vi "Proyecto Autotrónica.vi"() -> ()   [LabVIEW 2025]
uses:
  <vilib>/MakerHub/LINX/Public/Peripherals/Analog/Analog Read 1 Chan.vi
  <vilib>/MakerHub/LINX/Public/Peripherals/Digital/Digital Read 1 Chan.vi
  <vilib>/MakerHub/LINX/Public/Peripherals/Analog/Analog Read N Chans.vi
  <vilib>/MakerHub/LINX/Public/Peripherals/Digital/Digital Read N Chans.vi
  <vilib>/MakerHub/LINX/Private/Local IO/LinxAnalogRead.vi
  <vilib>/MakerHub/LINX/Public/Utilities/Check Channel.vi
  <vilib>/MakerHub/LINX/Private/Local IO/LinxDigitalRead.vi
  <vilib>/MakerHub/LINX/Public/Utilities/Open Serial.vi
  <vilib>/MakerHub/LINX/Private/Utilties/Generate Error.vi
  <vilib>/express/express shared/transition.llb/Dynamic To Waveform Array.vi
  <vilib>/express/express signal manip/GetorSetDDTAttributes/Set DDT Attributes/SetT0.vi
  <vilib>/express/express shared/transition.llb/Waveform Array To Dynamic.vi
  <vilib>/express/express signal manip/GetorSetDDTAttributes/Set DDT Attributes/Set DDT Properties.xnode
  <vilib>/MakerHub/LINX/LMH-LINX.lvlib
panel:
  out "?":bool
  out "?":bool
  out "?":bool
  out "?":bool
  out "Llave":bool
  out "Velocidad (MPH)":dbl
  in  "Serial Port":refnum<visa-resource-name>="N/A"
  out "TPMS":T1(graph)
  in  "stop":bool
  out "P3":bool
  out "P2":bool
  out "P1":bool
  out "Rueda RR ( BAR)":dbl
  out "Rueda RR  (PSI)":dbl
  out "Rueda LR (BAR)":dbl
  out "Rueda LR  (PSI)":dbl
  out "Rueda RF  (BAR)":dbl
  out "Rueda LF  (BAR)":dbl
  out "Rueda RF  (PSI)":dbl
  out "Rueda LF (PSI)":dbl
  out "Velocidad (km/h)":dbl(knob) scale=0.0..220.0
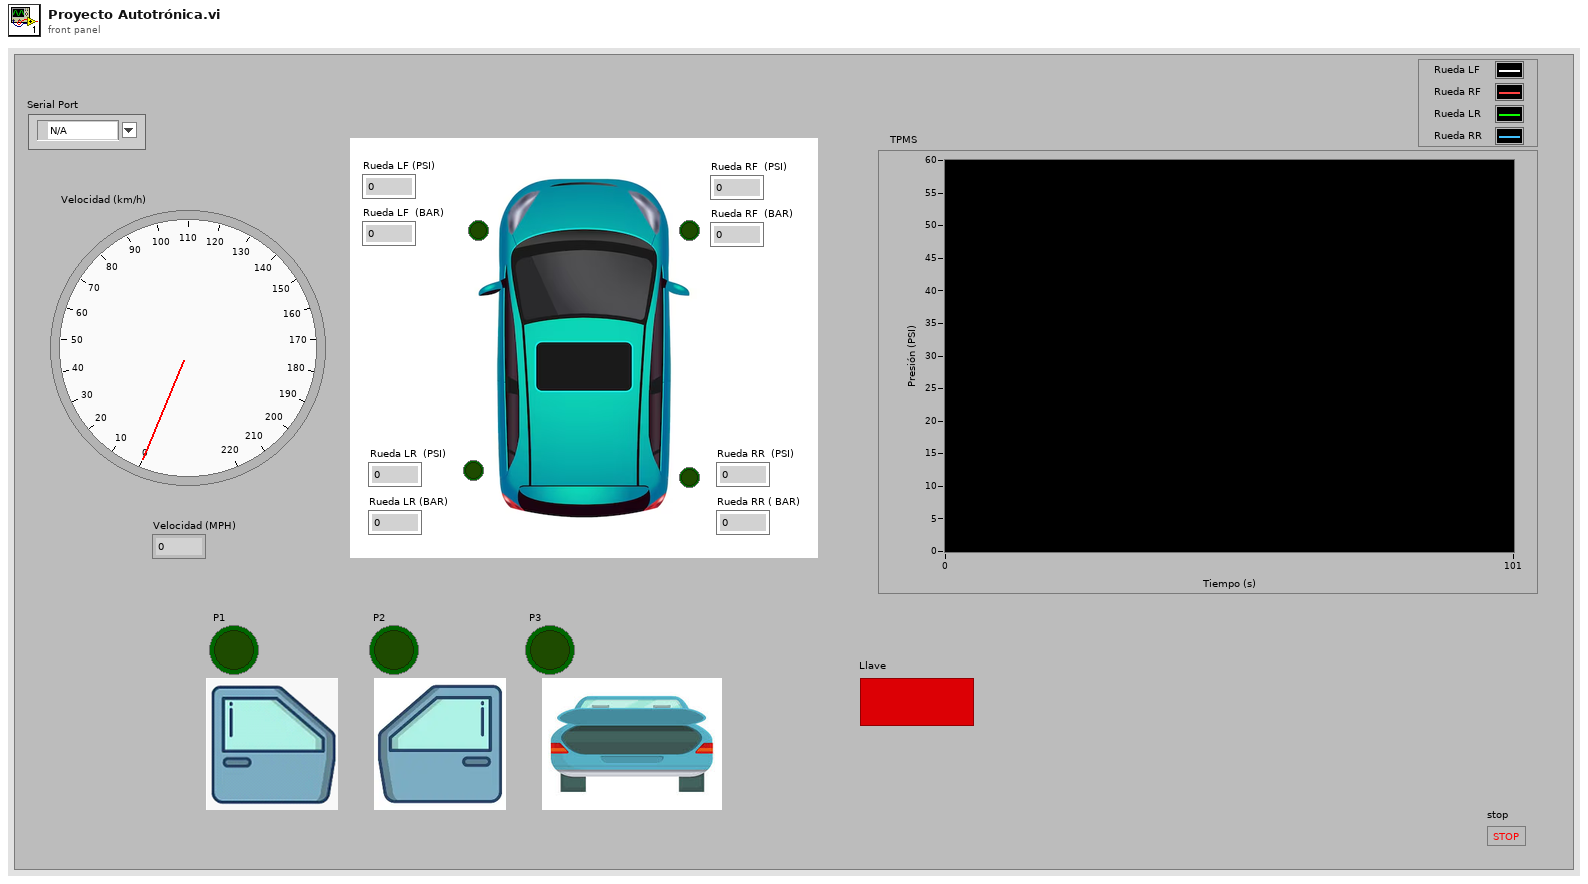
[diagram p1: front panel]
types:
  T1 = cluster{"Voltage":dbl, "Voltage":dbl, "Voltage":dbl, "Voltage":dbl}
  T2 = typedef "LMH-LINX.lvlib/LINX Ref.ctl" = cluster{"IO":T3, "Interface":T4, "LINX Device Config":T5}
  T3 = typedef "LMH-LINX.lvlib/Platform.ctl" = enum16{"Remote", "Local"}
  T4 = typedef "LMH-LINX.lvlib/Interface.ctl" = enum16{"Serial", "TCP"}
  T5 = typedef "LMH-LINX.lvlib/Device.lvlib/LINX Device Config.ctl" = cluster{"Interface":T4, "COM Port":refnum<visa-resource-name>, "TCP Configuration":T6, "Device Family":u8, "Device ID":u8, "Device Name":string, "TCP Ref":refnum<k5>, "Channels":T7}
  T6 = typedef "LMH-LINX.lvlib/Device.lvlib/TCP Config.ctl" = cluster{"IP Address":string, "Port":u16}
  T7 = typedef "LMH-LINX.lvlib/Channels.ctl" = cluster{"DI":u8[], "DO":u8[], "AI":u8[], "AO":u8[], "PWM":u8[], "QE":u8[], "UART":u8[], "I2C 2":u8[], "SPI":u8[], "CAN":u8[], "Servo":u8[], "AI Ref (V)":dbl, "AI Resolution (Bits)":u8, "AO Ref (V)":dbl, "AO Resolution (Bits)":u8}
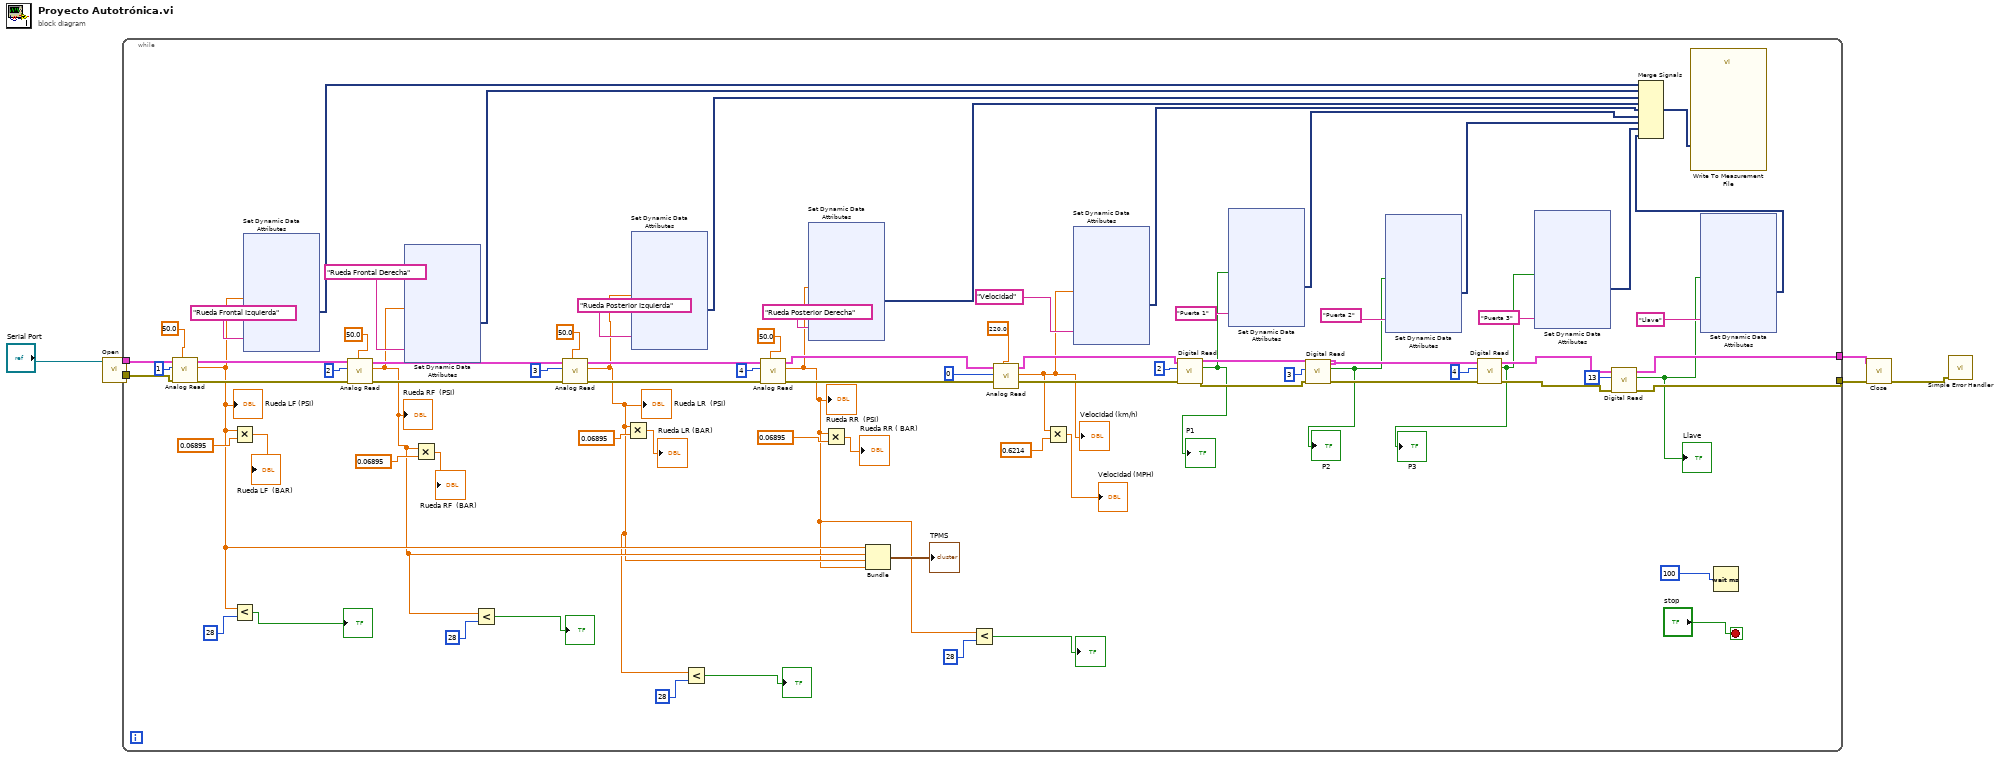
[diagram p0: block diagram]
diagram:
  n1 = call-poly <vilib>:"Open.vi"("Serial Port"="Serial Port") -> ("Error Out"=w3:errorcluster, "LINX Resource"=w6:T2)  [unwired: 8 in, 1 out]
  n2 = while {
    tunnel: w6 -> [w77]
    tunnel: [w28] -> w5
    tunnel: [w26] -> w4
    tunnel: w3 -> [w70]
    stop <- "stop" stop-if-true
    n3 = call-poly <vilib>:"Analog Read.vi"("Analog Ref Override (V)"=50.0, "Error In"=w70, "Analog Channel"=1, "LINX Resource"=w77) -> ("Error Out"=w71:errorcluster, "Voltage"=w18:dbl, "LINX Resource"=w76:T2)  [unwired: 4 in, 1 out]
    "Rueda LF (PSI)" <- w18
    n4 = Multiply(x=w18, y=0.06895) -> (x*y=→"Rueda LF  (BAR)":dbl)
    n5 = Less?(x=w18, y=28) -> (x < y?=→"?":bool)
    n6 = xnode "Set Dynamic Data Attributes"("Signals In"=w18, "Signal Name"="Rueda Frontal Izquierda") -> ("Signals Out"=w41:dynamicdata)  [unwired: 2 in, 1 out]
    n7 = call-poly <vilib>:"Analog Read.vi"("Analog Ref Override (V)"=50.0, "Error In"=w71, "Analog Channel"=2, "LINX Resource"=w76) -> ("Error Out"=w72:errorcluster, "Voltage"=w14:dbl, "LINX Resource"=w75:T2)  [unwired: 4 in, 1 out]
    "Rueda RF  (PSI)" <- w14
    n8 = xnode "Set Dynamic Data Attributes"("Signals In"=w14, "Signal Name"="Rueda Frontal Derecha") -> ("Signals Out"=w40:dynamicdata)  [unwired: 2 in, 1 out]
    n9 = Multiply(x=w14, y=0.06895) -> (x*y=→"Rueda RF  (BAR)":dbl)
    n10 = Less?(x=w14, y=28) -> (x < y?=→"?":bool)
    n11 = call-poly <vilib>:"Analog Read.vi"("Analog Ref Override (V)"=50.0, "Error In"=w72, "Analog Channel"=3, "LINX Resource"=w75) -> ("Error Out"=w73:errorcluster, "Voltage"=w11:dbl, "LINX Resource"=w74:T2)  [unwired: 4 in, 1 out]
    "Rueda LR  (PSI)" <- w11
    n12 = Multiply(x=w11, y=0.06895) -> (x*y=→"Rueda LR (BAR)":dbl)
    n13 = xnode "Set Dynamic Data Attributes"("Signals In"=w11, "Signal Name"="Rueda Posterior Izquierda") -> ("Signals Out"=w39:dynamicdata)  [unwired: 2 in, 1 out]
    n14 = Less?(x=w11, y=28) -> (x < y?=→"?":bool)
    n15 = call-poly <vilib>:"Analog Read.vi"("Analog Ref Override (V)"=50.0, "Error In"=w73, "Analog Channel"=4, "LINX Resource"=w74) -> ("Error Out"=w52:errorcluster, "Voltage"=w10:dbl, "LINX Resource"=w65:T2)  [unwired: 4 in, 1 out]
    "Rueda RR  (PSI)" <- w10
    n16 = xnode "Set Dynamic Data Attributes"("Signals In"=w10, "Signal Name"="Rueda Posterior Derecha") -> ("Signals Out"=w34:dynamicdata)  [unwired: 2 in, 1 out]
    n17 = Multiply(x=w10, y=0.06895) -> (x*y=→"Rueda RR ( BAR)":dbl)
    n18 = Bundle("Voltage"=w18, "Voltage"=w14, "Voltage"=w11, "Voltage"=w10) -> (→"TPMS":T1)  [unwired: 1 in]
    n19 = Less?(x=w10, y=28) -> (x < y?=→"?":bool)
    n20 = call-poly <vilib>:"Analog Read.vi"("Analog Ref Override (V)"=220.0, "Analog Channel"=0, "LINX Resource"=w65) -> ("Voltage"=w31:dbl, "LINX Resource"=w53:T2)  [unwired: 5 in, 2 out]
    "Velocidad (km/h)" <- w31
    n21 = Multiply(x=w31, y=0.6214) -> (x*y=→"Velocidad (MPH)":dbl)
    n22 = xnode "Set Dynamic Data Attributes"("Signals In"=w31, "Signal Name"="Velocidad") -> ("Signals Out"=w35:dynamicdata)  [unwired: 2 in, 1 out]
    n23 = call-poly <vilib>:"Digital Read.vi"("Error In"=w52, "DI Channel"=2, "LINX Resource"=w53) -> ("Error Out"=w50:errorcluster, "DI Value"=w21:bool, "LINX Resource"=w51:T2)  [unwired: 6 in]
    "P1" <- w21
    n24 = xnode "Set Dynamic Data Attributes"("Signals In"=w21, "Signal Name"="Puerta 1") -> ("Signals Out"=w36:dynamicdata)  [unwired: 2 in, 1 out]
    n25 = call-poly <vilib>:"Digital Read.vi"("Error In"=w50, "DI Channel"=3, "LINX Resource"=w51) -> ("Error Out"=w49:errorcluster, "DI Value"=w20:bool, "LINX Resource"=w48:T2)  [unwired: 6 in]
    "P2" <- w20
    n26 = xnode "Set Dynamic Data Attributes"("Signals In"=w20, "Signal Name"="Puerta 2") -> ("Signals Out"=w37:dynamicdata)  [unwired: 2 in, 1 out]
    n27 = call-poly <vilib>:"Digital Read.vi"("Error In"=w49, "DI Channel"=4, "LINX Resource"=w48) -> ("Error Out"=w27:errorcluster, "DI Value"=w19:bool, "LINX Resource"=w29:T2)  [unwired: 6 in]
    "P3" <- w19
    n28 = xnode "Set Dynamic Data Attributes"("Signals In"=w19, "Signal Name"="Puerta 3") -> ("Signals Out"=w38:dynamicdata)  [unwired: 2 in, 1 out]
    n29 = call-poly <vilib>:"Digital Read.vi"("Error In"=w27, "DI Channel"=13, "LINX Resource"=w29) -> ("Error Out"=w26:errorcluster, "DI Value"=w24:bool, "LINX Resource"=w28:T2)  [unwired: 6 in]
    "Llave" <- w24
    n30 = xnode "Set Dynamic Data Attributes"("Signals In"=w24, "Signal Name"="Llave") -> ("Signals Out"=w22:dynamicdata)  [unwired: 2 in, 1 out]
    n31 = Merge Signals(w41, w40, w39, w34, w35, w36, w37, w38, w22) -> (w33:dynamicdata)
    n32 = call "Write To Measurement File"("Signals"=w33) -> ()  [unwired: 16 in, 3 out]
    n33 = Wait (ms)(milliseconds to wait=100) -> ()  [unwired: 1 out]
  }
  n34 = call <vilib>:"Close.vi"("Error In"=w4, "LINX Resource"=w5) -> ("Error Out"=w1:errorcluster)  [unwired: 9 in]
  n35 = call <vilib>:"Simple Error Handler.vi"("error in (no error)"=w1) -> ()  [unwired: 4 in, 5 out]
